vi "Periodic Tasks.vi"(8 "error in":errorcluster) -> ()   [LabVIEW 2019]
doc: "This VI runs in parallel to other tasks. It can contain as many user-defined periodic loops as you need. These can carry out PID or other sorts of timed response."
uses:
  <vilib>/Rock Robotics/WPI/Utilities/WPI_GetSetVariantRefNum.vi
  <vilib>/Rock Robotics/Network Tables/NT Read Boolean.vi
  <vilib>/Rock Robotics/Network Tables/NT Write Number.vi
  Robot Global Data.vi
  <vilib>/Rock Robotics/WPI/RobotDrive/WPI_RobotDriveArcadeDrive_Standard(NoSaturation).vi
  <vilib>/Rock Robotics/Network Tables/NT Read Number.vi
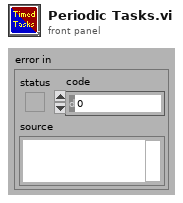
[diagram p1: front panel]
types:
  T1 = typedef "WPI_JoystickDevRef.ctl" = cluster{"Device":T2}
  T2 = typedef "WPI_JoystickDeviceEnum.ctl" = enum16{"USB 0", "USB 1", "USB 2", "USB 3", "USB 4", "USB 5"}
  T3 = typedef "WPI_RobotDriveDevRef.ctl" = cluster{"DevStatus":errorcluster, "Motors[]":T4[], "Square Inputs":bool, "Max Output":dbl}
  T4 = typedef "WPI_MotorControlDeviceRef.ctl" = cluster{"DeviceStatus":errorcluster, "Type":T5, "PWM":cluster{"PWM Channel":T6, "DeadBand":T7}, "CAN":cluster{"Device Number":u8, "SetOutput VI Ref":variant, "GetOutput VI Ref":variant, "Enable VI Ref":variant, "Disable VI Ref":variant, "Data":variant}, "Invert":bool, "DIO PWM":cluster{"PWM \"Enable\" Channel":T6, "DIOChannel":T8, "PWM Rate":dbl}}
  T5 = typedef "WPI_MotorControlType.ctl" = enum16{"PWM", "CAN", "DIO PWM"}
  T6 = typedef "FPGA_DIOPWMChannel.ctl" = enum8{"PWM 0", "PWM 1", "PWM 2", "PWM 3", "PWM 4", "PWM 5", "PWM 6", "PWM 7", "PWM 8", "PWM 9", "PWM MXP 0", "PWM MXP 1", "PWM MXP 2", "PWM MXP 3", "PWM MXP 4", "PWM MXP 5", "PWM MXP 6", "PWM MXP 7", "PWM MXP 8", "PWM MXP 9", "Invalid"}
  T7 = typedef "WPI_PWMDeadband.ctl" = cluster{"Name":string, "maxPositivePwm":i32, "minPositivePwm":i32, "centerPwm":i32, "maxNegativePwm":i32, "minNegativePwm":i32, "angularRange":u16}
  T8 = typedef "FPGA_DIOChannel.ctl" = enum8{"DIO 0", "DIO 1", "DIO 2", "DIO 3", "DIO 4", "DIO 5", "DIO 6", "DIO 7", "DIO 8", "DIO 9", "DIO MXP 0", "DIO MXP 1", "DIO MXP 2", "DIO MXP 3", "DIO MXP 4", "DIO MXP 5", "DIO MXP 6", "DIO MXP 7", "DIO MXP 8", "DIO MXP 9", "DIO MXP 10", "DIO MXP 11", "DIO MXP 12", "DIO MXP 13", "DIO MXP 14", "DIO MXP 15", "SPI Port CS1", "SPI Port CS2", "SPI Port CS3", "SPI Port MISO", "SPI Port MOSI", "Invalid"}
  T9 = cluster{"JoystickDevRef":T1, "RobotDriveDevRef":T3}
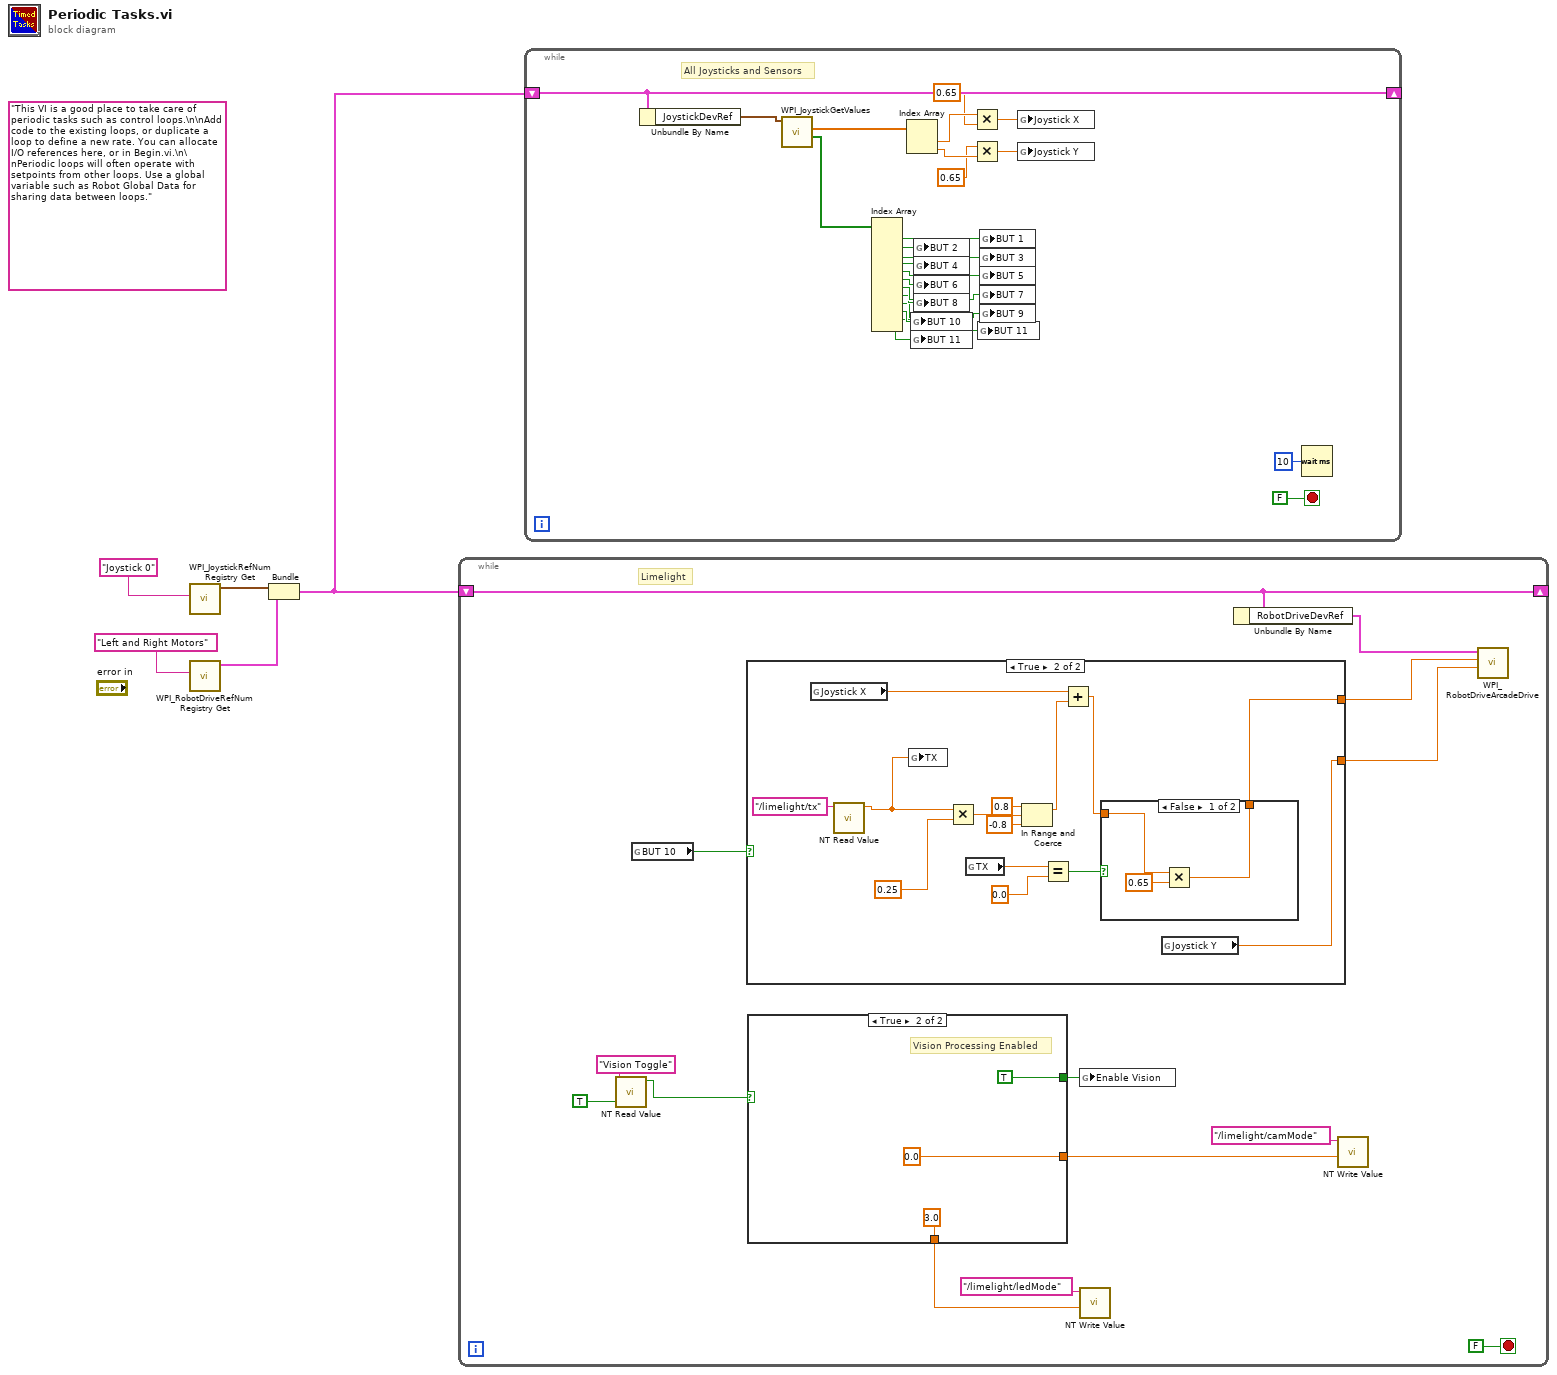
[diagram p0: block diagram]
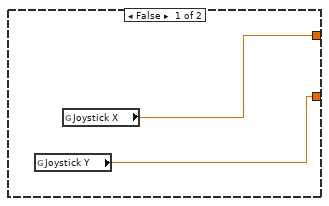
[diagram p2: hidden frame]
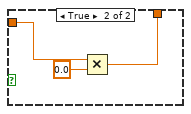
[diagram p3: hidden frame]
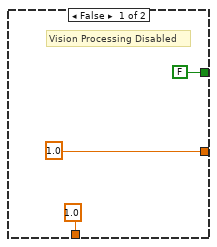
[diagram p4: hidden frame]
diagram:
  (unwired) "This VI is a good place to take care of periodic tasks such as control loops.\n\nAdd code to the existing loops, or duplicate a loop to define a new rate. You can allocate I/O references here, or in Begin.vi.\n\nPeriodic loops will often operate with setpoints from other loops. Use a global variable such as Robot Global Data for sharing data between loops."
  n1 = call <vilib>:"WPI_JoystickRefNum Registry Get.vi"("refnum name"="Joystick 0") -> ("JoystickDevRef"=w3:T1)  [unwired: 1 in, 9 out]
  n2 = call <vilib>:"WPI_RobotDriveRefNum Registry Get.vi"("refnum name"="Left and Right Motors") -> ("RobotDriveDevRef"=w2:T3)  [unwired: 1 in, 9 out]
  n3 = Bundle("JoystickDevRef"=w3, "RobotDriveDevRef"=w2) -> (w1:T9)  [unwired: 1 out]
  n4 = while {
    shift-right: [w15] -> _
    shift-left: w1 -> [w15]
    stop <- FALSE stop-if-true
    # "Limelight"
    n5 = call-poly <vilib>:"NT Read Value.vi"("Default Value"=TRUE, "Name"="Vision Toggle") -> ("Boolean"=w9:bool)  [unwired: 8 in, 1 out]
    n6 = global read "Robot Global Data.vi" "BUT 10"() -> (w6:bool)
    n7 = case shown="True" w6 {
      tunnel: [w21 w26] -> w16
      tunnel: [w20 w22] -> w7
      frame False {
        n8 = global read "Robot Global Data.vi" "Joystick Y"() -> (w20:dbl)
        n9 = global read "Robot Global Data.vi" "Joystick X"() -> (w21:dbl)
      }
      frame True {
        n10 = global read "Robot Global Data.vi" "Joystick X"() -> (w34:dbl)
        n11 = call-poly <vilib>:"NT Read Value.vi"("Name"="/limelight/tx") -> ("Numeric"=w28:dbl)  [unwired: 9 in, 1 out]
        n12 = global write "Robot Global Data.vi" "TX"(w28) -> ()
        n13 = Multiply(x=w28, y=0.25) -> (x*y=w32:dbl)
        n14 = global read "Robot Global Data.vi" "TX"() -> (w24:dbl)
        n15 = In Range and Coerce(upper limit=0.8, x=w32, lower limit=-0.8) -> (coerced(x)=w33:dbl)  [unwired: 1 out]
        n16 = Equal?(x=w24, y=0.0) -> (x = y?=w25:bool)
        n17 = Add(x=w34, y=w33) -> (x+y=w27:dbl)
        n18 = case shown="False" w25 {
          tunnel: w27 -> [w37 w41]
          tunnel: [w38 w39] -> w26
          frame False {
            n19 = Multiply(x=w37, y=0.65) -> (x*y=w38:dbl)
          }
          frame True {
            n20 = Multiply(x=w41, y=0.0) -> (x*y=w39:dbl)
          }
        }
        n21 = global read "Robot Global Data.vi" "Joystick Y"() -> (w22:dbl)
      }
    }
    n22 = case shown="True" w9 {
      tunnel: [FALSE ("Enable Vision") TRUE ("Enable Vision")] -> w18
      tunnel: [1.0 ("Numeric") 0.0 ("Numeric")] -> w13
      tunnel: [1.0 ("Numeric") 3.0 ("Numeric")] -> w10
      frame False {
        # "Vision Processing Disabled"
      }
      frame True {
        # "Vision Processing Enabled"
      }
    }
    n23 = global write "Robot Global Data.vi" "Enable Vision"(w18) -> ()
    n24 = call-poly <vilib>:"NT Write Value.vi"("Numeric"=w10, "Name"="/limelight/ledMode") -> ()  [unwired: 9 in, 1 out]
    n25 = Unbundle By Name(w15) -> ("RobotDriveDevRef"=w17:T3)
    n26 = call-poly <vilib>:"NT Write Value.vi"("Numeric"=w13, "Name"="/limelight/camMode") -> ()  [unwired: 9 in, 1 out]
    n27 = call-poly <vilib>:"WPI_RobotDriveArcadeDrive.vi"("Y axis value"=w7, "X axis value"=w16, "RobotDriveDevRef"=w17) -> ()  [unwired: 6 in, 3 out]
  }
  n28 = while {
    shift-right: [w70] -> _
    shift-left: w1 -> [w70]
    stop <- FALSE stop-if-true
    # "All Joysticks and Sensors"
    n29 = Unbundle By Name(w70) -> ("JoystickDevRef"=w68:T1)
    n30 = call <vilib>:"WPI_JoystickGetValues.vi"("JoystickDevRef"=w68) -> ("Buttons"=w60:bool[], "Axes"=w67:dbl[])  [unwired: 6 in, 3 out]
    n31 = Index Array(array=w60) -> (element #1=w59:bool, element #2=w58:bool, element #3=w57:bool, element #4=w56:bool, element #5=w55:bool, element #6=w54:bool, element #7=w53:bool, element #8=w52:bool, element #9=w51:bool, element #10=w50:bool, element #11=w49:bool, element #12=w48:bool)  [unwired: 12 in]
    n32 = Index Array(array=w67) -> (element #1=w66:dbl, element #2=w64:dbl)  [unwired: 2 in]
    n33 = global write "Robot Global Data.vi" "BUT 10"(w50) -> ()
    n34 = global write "Robot Global Data.vi" "BUT 11"(w48) -> ()
    n35 = global write "Robot Global Data.vi" "BUT 2"(w58) -> ()
    n36 = global write "Robot Global Data.vi" "BUT 4"(w56) -> ()
    n37 = global write "Robot Global Data.vi" "BUT 6"(w54) -> ()
    n38 = global write "Robot Global Data.vi" "BUT 8"(w52) -> ()
    n39 = Multiply(x=w66, y=0.65) -> (x*y=w62:dbl)
    n40 = Multiply(x=0.65, y=w64) -> (x*y=w61:dbl)
    n41 = global write "Robot Global Data.vi" "BUT 11"(w49) -> ()
    n42 = global write "Robot Global Data.vi" "BUT 1"(w59) -> ()
    n43 = global write "Robot Global Data.vi" "BUT 3"(w57) -> ()
    n44 = global write "Robot Global Data.vi" "BUT 5"(w55) -> ()
    n45 = global write "Robot Global Data.vi" "BUT 7"(w53) -> ()
    n46 = global write "Robot Global Data.vi" "BUT 9"(w51) -> ()
    n47 = global write "Robot Global Data.vi" "Joystick X"(w62) -> ()
    n48 = global write "Robot Global Data.vi" "Joystick Y"(w61) -> ()
    n49 = Wait (ms)(milliseconds to wait=u32 10) -> ()  [unwired: 1 out]
  }
